vi "lijnsensor.vi"() -> ()   [LabVIEW 2019]
panel:
  out "motor  zeer sterk links sneller 2":bool
  out "motor zwak naar rechts sneller  2":bool
  out "motor zeer sterk rechts sneller  2":bool
  out "motor zwak links sneller   2":bool
  out "motor naar links sneller  2":bool
  out "motor sterk rechts sneller   2":bool
  out "motoren sterk links sneller 2":bool
  out "motor naar rechts sneller 2":bool
  out "motor  stilleggen 2":bool
  in  "input array   3":dbl[](array[numeric])
  out "Numeric":i32
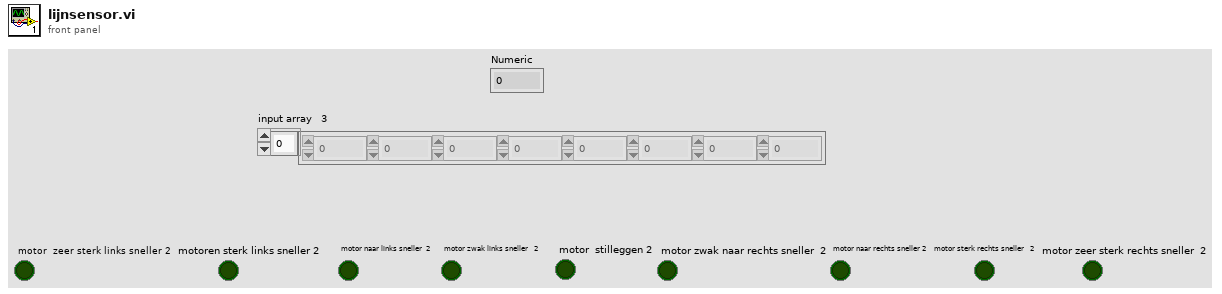
[diagram p1: front panel]
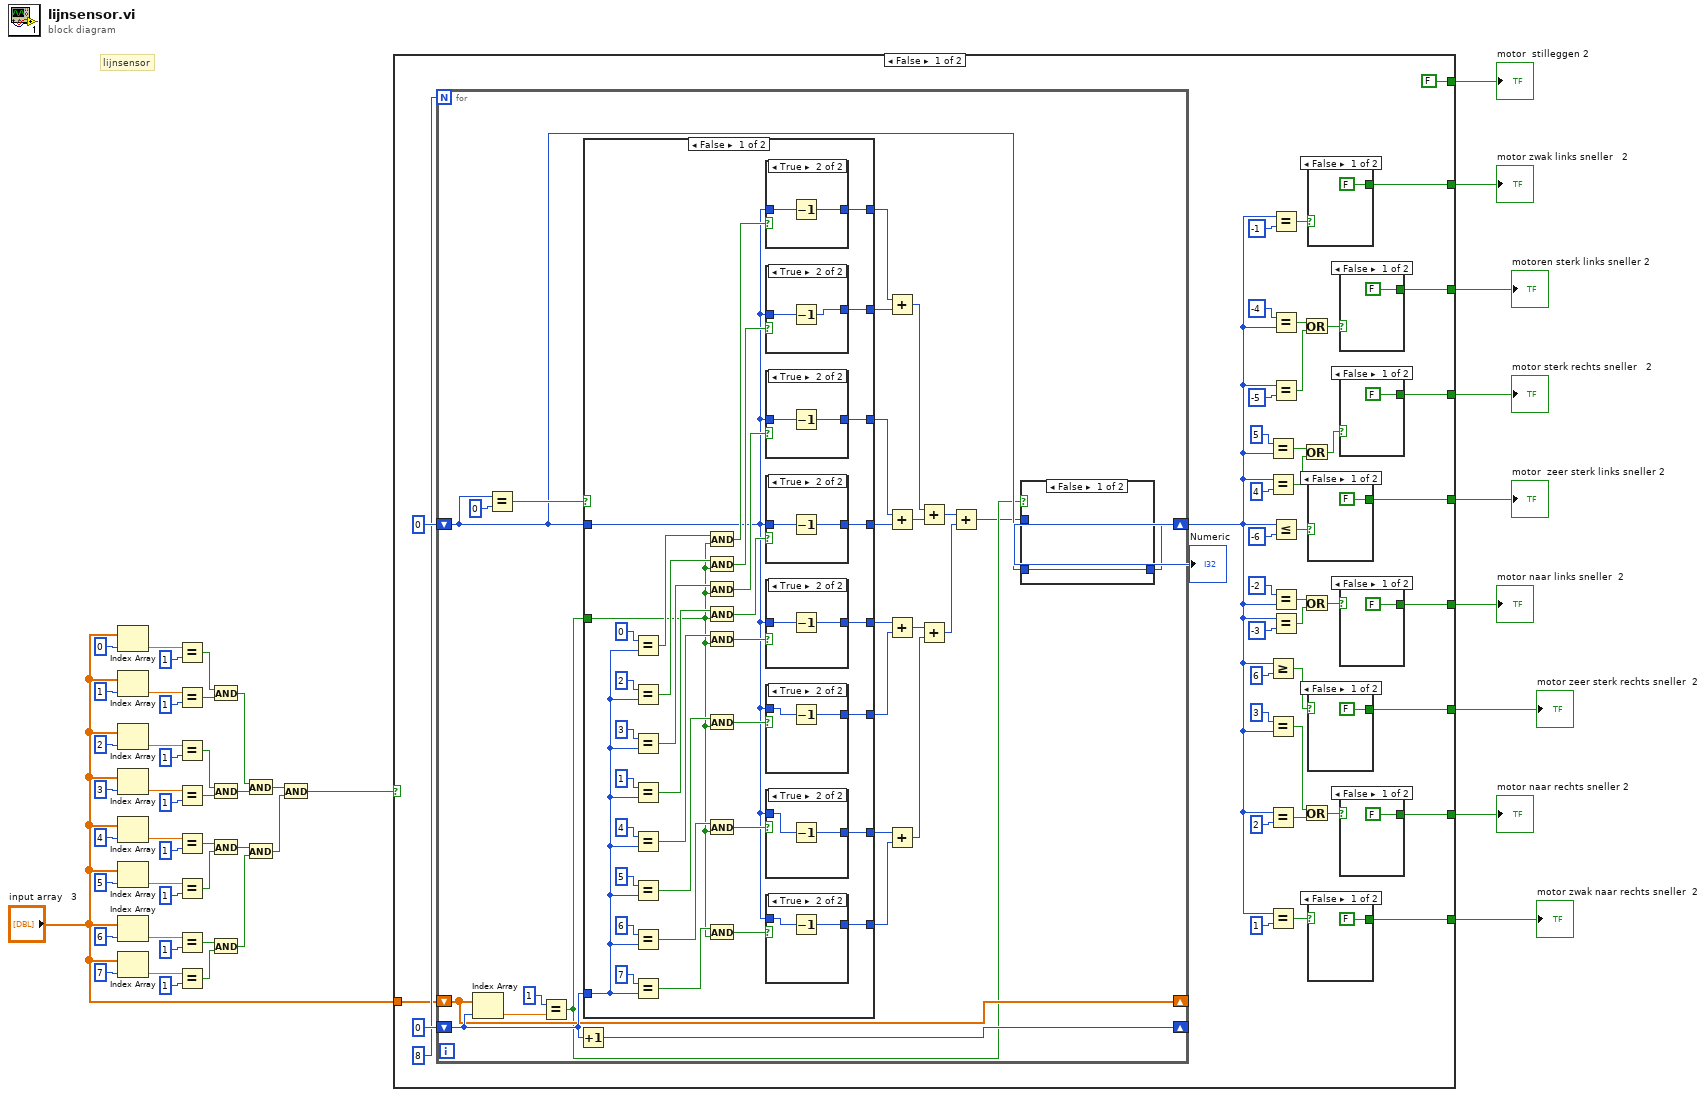
[diagram p0: block diagram]
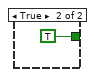
[diagram p2: hidden frame]
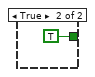
[diagram p3: hidden frame]
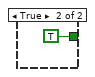
[diagram p4: hidden frame]
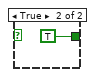
[diagram p5: hidden frame]
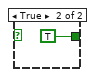
[diagram p6: hidden frame]
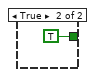
[diagram p7: hidden frame]
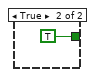
[diagram p8: hidden frame]
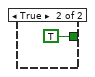
[diagram p9: hidden frame]
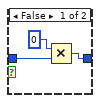
[diagram p11: hidden frame]
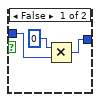
[diagram p12: hidden frame]
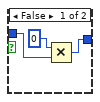
[diagram p13: hidden frame]
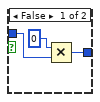
[diagram p14: hidden frame]
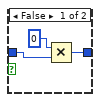
[diagram p15: hidden frame]
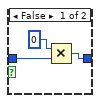
[diagram p16: hidden frame]
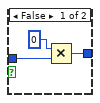
[diagram p17: hidden frame]
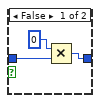
[diagram p18: hidden frame]
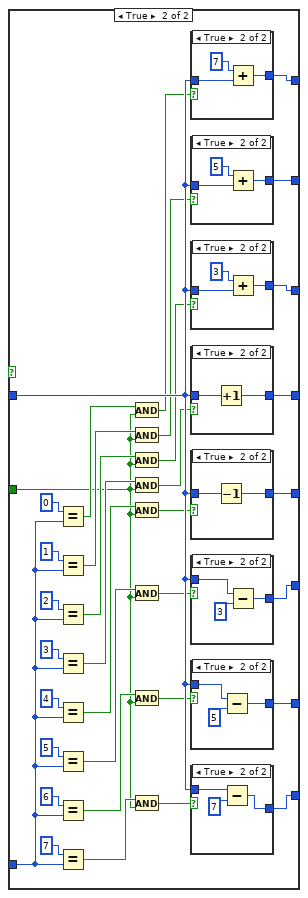
[diagram p19: hidden frame]
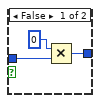
[diagram p20: hidden frame]
diagram:
  # "lijnsensor"
  n1 = Index Array(array="input array   3", index=0) -> (element=w28:dbl)
  n2 = Index Array(array="input array   3", index=1) -> (element=w49:dbl)
  n3 = Index Array(array="input array   3", index=2) -> (element=w43:dbl)
  n4 = Index Array(array="input array   3", index=3) -> (element=w46:dbl)
  n5 = Index Array(array="input array   3", index=4) -> (element=w40:dbl)
  n6 = Index Array(array="input array   3", index=5) -> (element=w37:dbl)
  n7 = Index Array(array="input array   3", index=6) -> (element=w34:dbl)
  n8 = Index Array(array="input array   3", index=7) -> (element=w31:dbl)
  n9 = Equal?(x=w28, y=1) -> (x = y?=w25:bool)
  n10 = Equal?(x=w49, y=1) -> (x = y?=w24:bool)
  n11 = Equal?(x=w43, y=1) -> (x = y?=w23:bool)
  n12 = Equal?(x=w46, y=1) -> (x = y?=w22:bool)
  n13 = Equal?(x=w40, y=1) -> (x = y?=w21:bool)
  n14 = Equal?(x=w37, y=1) -> (x = y?=w20:bool)
  n15 = Equal?(x=w34, y=1) -> (x = y?=w19:bool)
  n16 = Equal?(x=w31, y=1) -> (x = y?=w18:bool)
  n17 = And(x=w25, y=w24) -> (x .and. y?=w17:bool)
  n18 = And(x=w23, y=w22) -> (x .and. y?=w16:bool)
  n19 = And(x=w21, y=w20) -> (x .and. y?=w15:bool)
  n20 = And(x=w19, y=w18) -> (x .and. y?=w14:bool)
  n21 = And(x=w17, y=w16) -> (x .and. y?=w13:bool)
  n22 = And(x=w15, y=w14) -> (x .and. y?=w12:bool)
  n23 = And(x=w13, y=w12) -> (x .and. y?=w11:bool)
  n24 = case shown="False" w11 {
    tunnel: "input array   3" -> [w60 _]
    tunnel: [FALSE ("Boolean 2") TRUE ("Boolean 2")] -> w9
    tunnel: [w58 FALSE ("Boolean 2")] -> w8
    tunnel: [w57 FALSE ("Boolean 2")] -> w7
    tunnel: [w56 FALSE ("Boolean 2")] -> w6
    tunnel: [w55 FALSE ("Boolean 2")] -> w5
    tunnel: [w54 FALSE ("Boolean 2")] -> w4
    tunnel: [w53 FALSE ("Boolean 2")] -> w3
    tunnel: [w52 FALSE ("Boolean 2")] -> w2
    tunnel: [w51 FALSE ("Boolean 2")] -> w1
    frame False {
      n25 = for {
        N: 8 -> [_]
        shift-right: [w118] -> _
        shift-left: 0 -> [w132]
        shift-right: [w110] -> w50
        shift-left: 0 -> [w111]
        shift-right: [w123] -> _
        shift-left: w60 -> [w123]
        n26 = Index Array(array=w123, index=w132) -> (element=w122:dbl)
        n27 = Equal?(x=w111, y=0) -> (x = y?=w119:bool)
        n28 = Equal?(x=1, y=w122) -> (x = y?=w109:bool)
        n29 = Increment(x=w132) -> (x+1=w118:i32)
        n30 = case shown="False" w119 {
          tunnel: w132 -> [w142 w228]
          tunnel: [w136 w227] -> w131
          tunnel: [w143 w226] -> w130
          tunnel: [w144 w225] -> w129
          tunnel: [w145 w224] -> w128
          tunnel: w111 -> [w135 w223]
          tunnel: w109 -> [w141 w214]
          tunnel: [w139 w213] -> w117
          tunnel: [w140 w212] -> w116
          tunnel: [w137 w211] -> w114
          tunnel: [w138 w210] -> w113
          frame False {
            n31 = Equal?(x=0, y=w142) -> (x = y?=w162:bool)
            n32 = Equal?(x=2, y=w142) -> (x = y?=w168:bool)
            n33 = Equal?(x=3, y=w142) -> (x = y?=w169:bool)
            n34 = Equal?(x=1, y=w142) -> (x = y?=w154:bool)
            n35 = Equal?(x=4, y=w142) -> (x = y?=w166:bool)
            n36 = Equal?(x=5, y=w142) -> (x = y?=w167:bool)
            n37 = Equal?(x=6, y=w142) -> (x = y?=w165:bool)
            n38 = Equal?(x=7, y=w142) -> (x = y?=w164:bool)
            n39 = And(x=w162, y=w141) -> (x .and. y?=w146:bool)
            n40 = And(x=w168, y=w141) -> (x .and. y?=w148:bool)
            n41 = And(x=w169, y=w141) -> (x .and. y?=w149:bool)
            n42 = And(x=w154, y=w141) -> (x .and. y?=w147:bool)
            n43 = And(x=w166, y=w141) -> (x .and. y?=w150:bool)
            n44 = And(x=w167, y=w141) -> (x .and. y?=w151:bool)
            n45 = And(x=w165, y=w141) -> (x .and. y?=w152:bool)
            n46 = And(x=w164, y=w141) -> (x .and. y?=w153:bool)
            n47 = case shown="True" w146 {
              tunnel: [w171 w174] -> w140
              tunnel: w135 -> [w170 w173]
              frame False {
                n48 = Multiply(x=0, y=w170) -> (x*y=w171:i32)
              }
              frame True {
                n49 = Decrement(x=w173) -> (x-1=w174:i32)
              }
            }
            n50 = case shown="True" w148 {
              tunnel: [w202 w203] -> w139
              tunnel: w135 -> [w201 w204]
              frame False {
                n51 = Multiply(x=0, y=w201) -> (x*y=w202:i32)
              }
              frame True {
                n52 = Decrement(x=w204) -> (x-1=w203:i32)
              }
            }
            n53 = case shown="True" w149 {
              tunnel: [w196 w199] -> w138
              tunnel: w135 -> [w195 w198]
              frame False {
                n54 = Multiply(x=0, y=w195) -> (x*y=w196:i32)
              }
              frame True {
                n55 = Decrement(x=w198) -> (x-1=w199:i32)
              }
            }
            n56 = case shown="True" w147 {
              tunnel: [w206 w209] -> w137
              tunnel: w135 -> [w205 w208]
              frame False {
                n57 = Multiply(x=0, y=w205) -> (x*y=w206:i32)
              }
              frame True {
                n58 = Decrement(x=w208) -> (x-1=w209:i32)
              }
            }
            n59 = case shown="True" w150 {
              tunnel: [w191 w194] -> w136
              tunnel: w135 -> [w190 w193]
              frame False {
                n60 = Multiply(x=0, y=w190) -> (x*y=w191:i32)
              }
              frame True {
                n61 = Decrement(x=w193) -> (x-1=w194:i32)
              }
            }
            n62 = case shown="True" w151 {
              tunnel: [w181 w184] -> w143
              tunnel: w135 -> [w180 w183]
              frame False {
                n63 = Multiply(x=0, y=w180) -> (x*y=w181:i32)
              }
              frame True {
                n64 = Decrement(x=w183) -> (x-1=w184:i32)
              }
            }
            n65 = case shown="True" w152 {
              tunnel: [w186 w189] -> w144
              tunnel: w135 -> [w185 w188]
              frame False {
                n66 = Multiply(x=0, y=w185) -> (x*y=w186:i32)
              }
              frame True {
                n67 = Decrement(x=w188) -> (x-1=w189:i32)
              }
            }
            n68 = case shown="True" w153 {
              tunnel: [w175 w179] -> w145
              tunnel: w135 -> [w176 w178]
              frame False {
                n69 = Multiply(x=0, y=w176) -> (x*y=w175:i32)
              }
              frame True {
                n70 = Decrement(x=w178) -> (x-1=w179:i32)
              }
            }
          }
          frame True {
            n71 = Equal?(x=0, y=w228) -> (x = y?=w237:bool)
            n72 = Equal?(x=1, y=w228) -> (x = y?=w229:bool)
            n73 = Equal?(x=2, y=w228) -> (x = y?=w243:bool)
            n74 = Equal?(x=3, y=w228) -> (x = y?=w244:bool)
            n75 = Equal?(x=4, y=w228) -> (x = y?=w241:bool)
            n76 = Equal?(x=5, y=w228) -> (x = y?=w242:bool)
            n77 = Equal?(x=6, y=w228) -> (x = y?=w240:bool)
            n78 = Equal?(x=7, y=w228) -> (x = y?=w239:bool)
            n79 = And(x=w237, y=w214) -> (x .and. y?=w215:bool)
            n80 = And(x=w229, y=w214) -> (x .and. y?=w216:bool)
            n81 = And(x=w243, y=w214) -> (x .and. y?=w217:bool)
            n82 = And(x=w244, y=w214) -> (x .and. y?=w218:bool)
            n83 = And(x=w241, y=w214) -> (x .and. y?=w219:bool)
            n84 = And(x=w242, y=w214) -> (x .and. y?=w220:bool)
            n85 = And(x=w240, y=w214) -> (x .and. y?=w221:bool)
            n86 = And(x=w239, y=w214) -> (x .and. y?=w222:bool)
            n87 = case shown="True" w215 {
              tunnel: w223 -> [w245 w249]
              tunnel: [w246 w248] -> w212
              frame False {
                n88 = Multiply(x=0, y=w245) -> (x*y=w246:i32)
              }
              frame True {
                n89 = Add(x=7, y=w249) -> (x+y=w248:i32)
              }
            }
            n90 = case shown="True" w216 {
              tunnel: w223 -> [w285 w288]
              tunnel: [w286 w289] -> w213
              frame False {
                n91 = Multiply(x=0, y=w285) -> (x*y=w286:i32)
              }
              frame True {
                n92 = Add(x=5, y=w288) -> (x+y=w289:i32)
              }
            }
            n93 = case shown="True" w217 {
              tunnel: w223 -> [w279 w283]
              tunnel: [w280 w282] -> w210
              frame False {
                n94 = Multiply(x=0, y=w279) -> (x*y=w280:i32)
              }
              frame True {
                n95 = Add(x=3, y=w283) -> (x+y=w282:i32)
              }
            }
            n96 = case shown="True" w218 {
              tunnel: w223 -> [w275 w278]
              tunnel: [w274 w277] -> w211
              frame False {
                n97 = Multiply(x=0, y=w275) -> (x*y=w274:i32)
              }
              frame True {
                n98 = Increment(x=w278) -> (x+1=w277:i32)
              }
            }
            n99 = case shown="True" w219 {
              tunnel: w223 -> [w269 w273]
              tunnel: [w270 w272] -> w227
              frame False {
                n100 = Multiply(x=0, y=w269) -> (x*y=w270:i32)
              }
              frame True {
                n101 = Decrement(x=w273) -> (x-1=w272:i32)
              }
            }
            n102 = case shown="True" w220 {
              tunnel: w223 -> [w258 w260]
              tunnel: [w257 w262] -> w226
              frame False {
                n103 = Multiply(x=0, y=w258) -> (x*y=w257:i32)
              }
              frame True {
                n104 = Subtract(x=w260, y=3) -> (x-y=w262:i32)
              }
            }
            n105 = case shown="True" w221 {
              tunnel: w223 -> [w264 w266]
              tunnel: [w263 w267] -> w225
              frame False {
                n106 = Multiply(x=0, y=w264) -> (x*y=w263:i32)
              }
              frame True {
                n107 = Subtract(x=w266, y=5) -> (x-y=w267:i32)
              }
            }
            n108 = case shown="True" w222 {
              tunnel: w223 -> [w251 w254]
              tunnel: [w252 w255] -> w224
              frame False {
                n109 = Multiply(x=0, y=w251) -> (x*y=w252:i32)
              }
              frame True {
                n110 = Subtract(x=w254, y=7) -> (x-y=w255:i32)
              }
            }
          }
        }
        n111 = Add(x=w116, y=w117) -> (x+y=w115:i32)
        n112 = Add(x=w113, y=w114) -> (x+y=w112:i32)
        n113 = Add(x=w131, y=w130) -> (x+y=w126:i32)
        n114 = Add(x=w129, y=w128) -> (x+y=w127:i32)
        n115 = Add(x=w115, y=w112) -> (x+y=w125:i32)
        n116 = Add(x=w126, y=w127) -> (x+y=w124:i32)
        n117 = Add(x=w125, y=w124) -> (x+y=w108:i32)
        n118 = case shown="False" w109 {
          tunnel: w111 -> [w133 _]
          tunnel: [w133 w134] -> w110
          tunnel: w108 -> [_ w134]
          frame False {
          }
          frame True {
          }
        }
      }
      "Numeric" <- w50
      n119 = Equal?(x=5, y=w50) -> (x = y?=w81:bool)
      n120 = Equal?(x=w50, y=4) -> (x = y?=w82:bool)
      n121 = Greater Or Equal?(x=w50, y=6) -> (x >= y?=w86:bool)
      n122 = Equal?(x=3, y=w50) -> (x = y?=w77:bool)
      n123 = Equal?(x=w50, y=2) -> (x = y?=w78:bool)
      n124 = Equal?(x=w50, y=1) -> (x = y?=w87:bool)
      n125 = Equal?(x=w50, y=-1) -> (x = y?=w65:bool)
      n126 = Equal?(x=-4, y=w50) -> (x = y?=w67:bool)
      n127 = Equal?(x=w50, y=-5) -> (x = y?=w68:bool)
      n128 = Less Or Equal?(x=w50, y=-6) -> (x <= y?=w63:bool)
      n129 = Equal?(x=-2, y=w50) -> (x = y?=w71:bool)
      n130 = Equal?(x=w50, y=-3) -> (x = y?=w72:bool)
      n131 = Or(x=w67, y=w68) -> (x .or. y?=w61:bool)
      n132 = Or(x=w81, y=w82) -> (x .or. y?=w83:bool)
      n133 = Or(x=w71, y=w72) -> (x .or. y?=w64:bool)
      n134 = Or(x=w77, y=w78) -> (x .or. y?=w75:bool)
      n135 = case shown="False" w65 {
        tunnel: [FALSE ("Boolean 2") TRUE ("Boolean 2")] -> w51
        frame False {
        }
        frame True {
        }
      }
      n136 = case shown="False" w63 {
        tunnel: [FALSE ("Boolean 2") TRUE ("Boolean 2")] -> w54
        frame False {
        }
        frame True {
        }
      }
      n137 = case shown="False" w86 {
        tunnel: [FALSE ("Boolean 2") TRUE ("Boolean 2")] -> w52
        frame False {
        }
        frame True {
        }
      }
      n138 = case shown="False" w87 {
        tunnel: [FALSE ("Boolean 2") TRUE ("Boolean 2")] -> w53
        frame False {
        }
        frame True {
        }
      }
      n139 = case shown="False" w61 {
        tunnel: [FALSE ("Boolean 2") TRUE ("Boolean 2")] -> w56
        frame False {
        }
        frame True {
        }
      }
      n140 = case shown="False" w83 {
        tunnel: [FALSE ("Boolean 2") TRUE ("Boolean 2")] -> w57
        frame False {
        }
        frame True {
        }
      }
      n141 = case shown="False" w64 {
        tunnel: [FALSE ("Boolean 2") TRUE ("Boolean 2")] -> w58
        frame False {
        }
        frame True {
        }
      }
      n142 = case shown="False" w75 {
        tunnel: [FALSE ("Boolean 2") TRUE ("Boolean 2")] -> w55
        frame False {
        }
        frame True {
        }
      }
    }
    frame True {
    }
  }
  "motor  stilleggen 2" <- w9
  "motor naar rechts sneller 2" <- w5
  "motoren sterk links sneller 2" <- w6
  "motor sterk rechts sneller   2" <- w7
  "motor naar links sneller  2" <- w8
  "motor zwak links sneller   2" <- w1
  "motor zeer sterk rechts sneller  2" <- w2
  "motor zwak naar rechts sneller  2" <- w3
  "motor  zeer sterk links sneller 2" <- w4
